vi "tdoa.vi"() -> ()   [LabVIEW 2015]
uses:
  <vilib>/rvi/Emulation/niFpgaGetClockAttributes.vi
  <vilib>/rvi/Emulation/niFpgaSctlEmulationGetInTimedLoop.vi
  <vilib>/rvi/Emulation/niFpgaEmulationReportErrorSimple.vi
  <vilib>/rvi/DataTransferAndStorage/Container/Common/niFpgaContainerGetUniqueNameForEmu.vi
  <vilib>/rvi/DataTransferAndStorage/Container/Common/niFpgaContainerSetEmuInfo.vi
  <vilib>/rvi/eio/common/nirviEmuReportErrorAndStop.vi
  <vilib>/rvi/eio/common/nirviEmuTemplateMethod_errors.vi
  <vilib>/rvi/interface/RandomDataEmulation/niFpgaRandomDataHandleErrors.vi
  <vilib>/rvi/DataTransferAndStorage/Container/Common/niFpgaContainerExecOnDevCompGetState.vi
  <vilib>/rvi/Emulation/niFpgaEmulationIsFPGAContextNoSignature.vi
  <vilib>/rvi/errors/niFpgaSetErrorForExecOnDevCompSimple.vi
  <vilib>/rvi/FIFO/Fifo_Resource/nirvififoEmulationSetSize.vi
  <vilib>/rvi/FIFO/Fifo_Resource/nirviFifoEmulationQueueMgr.vi
  <instcachedir>/0/nirviFifoEmulationQueueMgr_E5CAEC123FF24DC58D834DCA3CDAA9B5.lvgen/nirviFifoEmulationQueueMgr_E5CAEC123FF24DC58D834DCA3CDAA9B5_010.vi
  <vilib>/rvi/FIFO/Fifo_Resource/nirvififoEmulationDetermineInputValidOut.vi
  <vilib>/rvi/FIFO/Fifo_Resource/nirvififoEmulationCreateLock.vi
  <vilib>/rvi/Emulation/niFpgaProcessEmulError.vi
  <vilib>/rvi/FIFO/Fifo_Resource/nirvififoEmulationObtainLock.vi
  <vilib>/rvi/FIFO/Fifo_Resource/nirvififoEmulationReleaseLock.vi
  <vilib>/rvi/occurrence/nirviWaitOnOccurrenceBase.vi
  <vilib>/rvi/errors/nirviReportUnexpectedCaseInternalError.vi
  <vilib>/rvi/errors/nirviReportUnexpectedCaseInternalError (U32).vi
  <vilib>/Utility/error.llb/Clear Errors.vi
  <instcachedir>/0/nirviFifoEmulationQueueMgr_E5CAEC123FF24DC58D834DCA3CDAA9B5.lvgen/nirviFifoEmulationQueueMgr_E5CAEC123FF24DC58D834DCA3CDAA9B5_011.vi
  <vilib>/rvi/Emulation/niFpgaCriticalErrorInLSC.vi
  <vilib>/rvi/Memory/Memory_Emulation/niFpgaMemoryEmulationCacheClearOnFirstRun.vi
  <vilib>/rvi/Memory/Memory_Emulation/nirvimemoryEmulationManagerCache_MakeExclusive.vi
  <vilib>/rvi/Memory/Memory_Emulation/niFpgaMemoryEmulationValidateCache.vi
  <vilib>/rvi/Memory/Memory_Emulation/nirvimemoryEmulationManagerCache_InsertValue.vi
  <vilib>/rvi/Memory/Memory_Emulation/nirvimemoryEmulationManagerCache_ReleaseExclusive.vi
  <vilib>/rvi/Memory/Memory_Emulation/nirvimemoryEmulationManagerCache_GetValue.vi
  <vilib>/rvi/Memory/Memory_Emulation/nirvimemoryEmulationManagerCache_SetValue.vi
  <vilib>/rvi/Emulation/niFpgaSctlEmulationResourceMgr.vi
  <vilib>/rvi/LocalResourceManager/LocalResourceManager.xnode
  <vilib>/eio/EIONode/EIONode.xnode
  <vilib>/rvi/DataTransferAndStorage/Container/XNode/niFpgaContainer.xnode
  <vilib>/rvi/interface/RandomDataEmulation/nirviRandomDataFpgaReadWriteTemplate.vi
  <vilib>/rvi/FIFO/Fifo_Resource/niFpgaFifoEmulationRefIn.vi
  <vilib>/rvi/Memory/Memory_Emulation/niFpgaMemoryEmulationRefIn.vi
panel:
  out "xcorr1":fxp<+/-,32,30>
  out "xcorr1":fxp<+/-,32,30>
  out "Numeric 3":i32
  out "Numeric 2":i32
  out "Numeric":i32
  out "xcorr0":fxp<+/-,32,30>
  out "tdoa0":i32
  out "tdoa1":i32
  out "tdoa2":i32
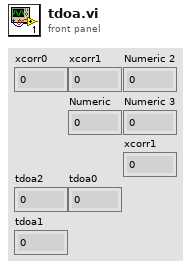
[diagram p1: front panel]
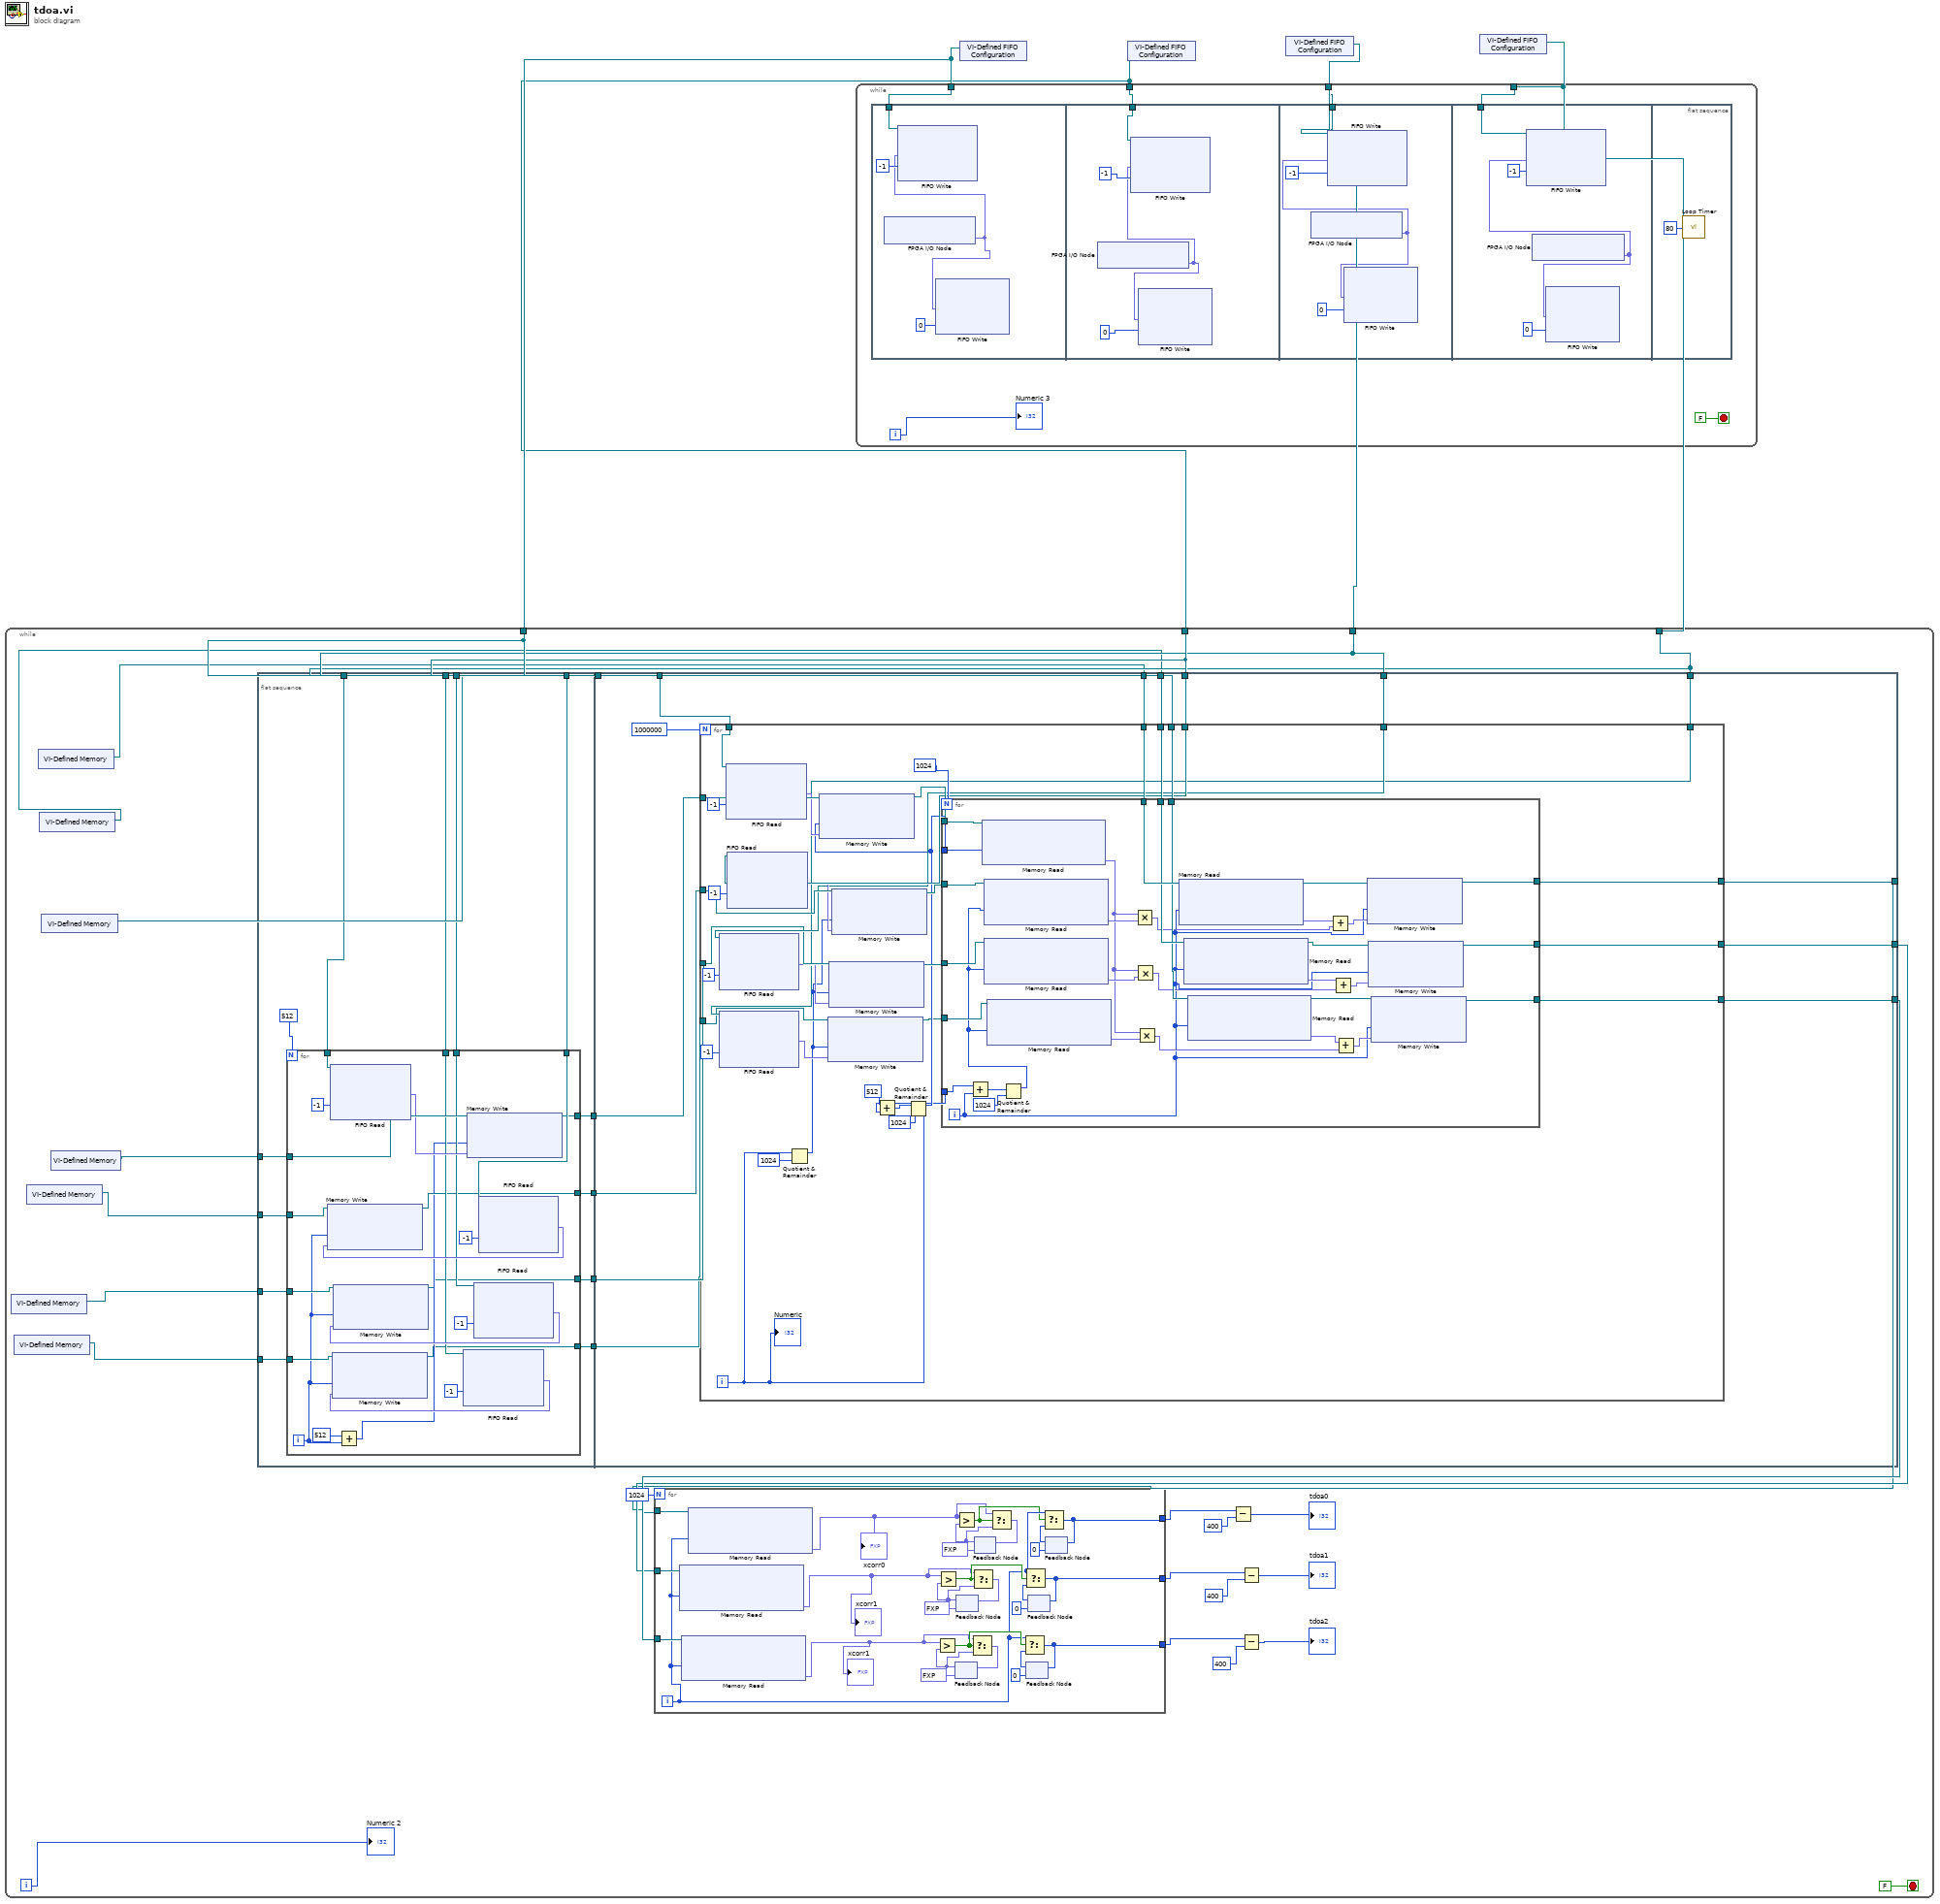
[diagram p0: block diagram]
diagram:
  n1 = xnode "VI-Defined FIFO Configuration"() -> ("FIFO Out"=w4:refnum<k21>)
  n2 = xnode "VI-Defined FIFO Configuration"() -> ("FIFO Out"=w3:refnum<k21>)
  n3 = xnode "VI-Defined FIFO Configuration"() -> ("FIFO Out"=w1:refnum<k21>)
  n4 = xnode "VI-Defined FIFO Configuration"() -> ("FIFO Out"=w2:refnum<k21>)
  n5 = while {
    tunnel: w1 -> [w30]
    tunnel: w2 -> [w29]
    tunnel: w4 -> [w33]
    tunnel: w3 -> [w31]
    i -> [w8]
    stop <- FALSE stop-if-true
    n6 = xnode "VI-Defined Memory"() -> ("Memory Out"=w6:refnum<k21>)
    n7 = xnode "VI-Defined Memory"() -> ("Memory Out"=w7:refnum<k21>)
    n8 = xnode "VI-Defined Memory"() -> ("Memory Out"=w5:refnum<k21>)
    n9 = xnode "VI-Defined Memory"() -> ("Memory Out"=w24:refnum<k21>)
    n10 = xnode "VI-Defined Memory"() -> ("Memory Out"=w23:refnum<k21>)
    n11 = xnode "VI-Defined Memory"() -> ("Memory Out"=w22:refnum<k21>)
    n12 = xnode "VI-Defined Memory"() -> ("Memory Out"=w32:refnum<k21>)
    n13 = flat-sequence {
      tunnel: w33 -> [w73]
      tunnel: w32 -> [w75]
      tunnel: w5 -> [w72]
      tunnel: w31 -> [w71]
      tunnel: w6 -> [w70]
      tunnel: w30 -> [w69]
      tunnel: w7 -> [w68]
      tunnel: w29 -> [w67]
      tunnel: [w66] -> w28
      tunnel: [w65] -> w27
      tunnel: [w64] -> w26
      tunnel: [w63] -> w25
      tunnel: w30 -> [w113]
      tunnel: w29 -> [w112]
      tunnel: w33 -> [w110]
      tunnel: w31 -> [w109]
      tunnel: w28 -> [w108]
      tunnel: w27 -> [w107]
      tunnel: w26 -> [w106]
      tunnel: w25 -> [w105]
      tunnel: w24 -> [w104]
      tunnel: w23 -> [w103]
      tunnel: w22 -> [w102]
      tunnel: [w101] -> w18
      tunnel: [w100] -> w17
      tunnel: [w99] -> w16
      frame #0 {
        n14 = for {
          N: 512 -> [_]
          tunnel: w75 -> [w98]
          tunnel: w73 -> [w97]
          tunnel: w72 -> [w94]
          tunnel: w71 -> [w92]
          tunnel: w70 -> [w89]
          tunnel: w69 -> [w88]
          tunnel: w68 -> [w85]
          tunnel: w67 -> [w84]
          tunnel: [w81] -> w66
          tunnel: [w80] -> w65
          tunnel: [w77] -> w64
          tunnel: [w76] -> w63
          i -> [w78]
          n15 = xnode ("FIFO Read")("Timeout"=-1, "FIFO In"=w97) -> ("Element"=w95:fxp<+/-,16,16>)  [unwired: 2 out]
          n16 = Add(x=512, y=w78) -> (x+y=w79:i32)
          n17 = xnode ("FIFO Read")("Timeout"=-1, "FIFO In"=w84) -> ("Element"=w83:fxp<+/-,32,16>)  [unwired: 2 out]
          n18 = xnode ("Memory Write")("Address"=w78, "Data"=w83, "Memory In"=w85) -> ("Memory Out"=w76:refnum<k21>)
          n19 = xnode ("Memory Write")("Address"=w79, "Data"=w95, "Memory In"=w98) -> ("Memory Out"=w81:refnum<k21>)
          n20 = xnode ("FIFO Read")("Timeout"=-1, "FIFO In"=w88) -> ("Element"=w87:fxp<+/-,32,16>)  [unwired: 2 out]
          n21 = xnode ("Memory Write")("Address"=w78, "Data"=w87, "Memory In"=w89) -> ("Memory Out"=w77:refnum<k21>)
          n22 = xnode ("FIFO Read")("Timeout"=-1, "FIFO In"=w92) -> ("Element"=w91:fxp<+/-,32,16>)  [unwired: 2 out]
          n23 = xnode ("Memory Write")("Address"=w78, "Data"=w91, "Memory In"=w94) -> ("Memory Out"=w80:refnum<k21>)
        }
      }
      frame #1 {
        n24 = for {
          N: 1000000 -> [_]
          tunnel: w113 -> [w131]
          tunnel: w112 -> [w124]
          tunnel: w110 -> [w138]
          tunnel: w109 -> [w135]
          tunnel: w108 -> [w140]
          tunnel: w107 -> [w134]
          tunnel: w106 -> [w128]
          tunnel: w105 -> [w123]
          tunnel: w104 -> [w143]
          tunnel: w103 -> [w142]
          tunnel: w102 -> [w141]
          tunnel: [w117] -> w101
          tunnel: [w116] -> w100
          tunnel: [w115] -> w99
          i -> [w114]
          n25 = xnode ("FIFO Read")("Timeout"=-1, "FIFO In"=w131) -> ("Element"=w125:fxp<+/-,32,16>)  [unwired: 2 out]
          n26 = xnode ("FIFO Read")("Timeout"=-1, "FIFO In"=w124) -> ("Element"=w121:fxp<+/-,32,16>)  [unwired: 2 out]
          n27 = xnode ("FIFO Read")("Timeout"=-1, "FIFO In"=w138) -> ("Element"=w136:fxp<+/-,16,16>)  [unwired: 2 out]
          n28 = xnode ("FIFO Read")("Timeout"=-1, "FIFO In"=w135) -> ("Element"=w132:fxp<+/-,32,16>)  [unwired: 2 out]
          n29 = Quotient & Remainder(x=w114, y=1024) -> (x-y*floor(x/y)=w118:i32)  [unwired: 1 out]
          n30 = xnode ("Memory Write")("Address"=w118, "Data"=w121, "Memory In"=w123) -> ("Memory Out"=w122:refnum<k21>)
          n31 = xnode ("Memory Write")("Address"=w118, "Data"=w125, "Memory In"=w128) -> ("Memory Out"=w127:refnum<k21>)
          n32 = xnode ("Memory Write")("Address"=w118, "Data"=w132, "Memory In"=w134) -> ("Memory Out"=w133:refnum<k21>)
          n33 = Add(x=512, y=w114) -> (x+y=w145:i32)
          n34 = Quotient & Remainder(x=w145, y=1024) -> (x-y*floor(x/y)=w126:i32)  [unwired: 1 out]
          n35 = xnode ("Memory Write")("Address"=w126, "Data"=w136, "Memory In"=w140) -> ("Memory Out"=w139:refnum<k21>)
          n36 = for {
            N: 1024 -> [_]
            tunnel: w139 -> [w179]
            tunnel: w133 -> [w178]
            tunnel: w114 -> [w176]
            tunnel: w126 -> [w177]
            tunnel: w127 -> [w173]
            tunnel: w122 -> [w172]
            tunnel: w143 -> [w166]
            tunnel: w142 -> [w165]
            tunnel: w141 -> [w164]
            tunnel: [w150] -> w115
            tunnel: [w149] -> w116
            tunnel: [w148] -> w117
            i -> [w151]
            n37 = Add(x=w176, y=w151) -> (x+y=w175:i32)
            n38 = xnode ("Memory Read")("Address"=w177, "Memory In"=w179) -> ("Data"=w167:fxp<+/-,32,16>)  [unwired: 1 out]
            n39 = Quotient & Remainder(x=w175, y=1024) -> (x-y*floor(x/y)=w171:i32)  [unwired: 1 out]
            n40 = xnode ("Memory Read")("Address"=w171, "Memory In"=w178) -> ("Data"=w168:fxp<+/-,32,16>)  [unwired: 1 out]
            n41 = xnode ("Memory Read")("Address"=w171, "Memory In"=w173) -> ("Data"=w169:fxp<+/-,32,16>)  [unwired: 1 out]
            n42 = xnode ("Memory Read")("Address"=w171, "Memory In"=w172) -> ("Data"=w170:fxp<+/-,32,16>)  [unwired: 1 out]
            n43 = Multiply(x=w167, y=w168) -> (x*y=w162:fxp<+/-,64,32>)
            n44 = Multiply(x=w167, y=w169) -> (x*y=w160:fxp<+/-,64,32>)
            n45 = Multiply(x=w167, y=w170) -> (x*y=w158:fxp<+/-,64,32>)
            n46 = xnode ("Memory Read")("Address"=w151, "Memory In"=w166) -> ("Data"=w163:fxp<+/-,64,32>, "Memory Out"=w157:refnum<k21>)
            n47 = xnode ("Memory Read")("Address"=w151, "Memory In"=w165) -> ("Data"=w161:fxp<+/-,64,32>, "Memory Out"=w156:refnum<k21>)
            n48 = xnode ("Memory Read")("Address"=w151, "Memory In"=w164) -> ("Data"=w159:fxp<+/-,64,32>, "Memory Out"=w155:refnum<k21>)
            n49 = Add(x=w163, y=w162) -> (x+y=w152:fxp<+/-,64,33>)
            n50 = Add(x=w161, y=w160) -> (x+y=w153:fxp<+/-,64,33>)
            n51 = Add(x=w159, y=w158) -> (x+y=w154:fxp<+/-,64,33>)
            n52 = xnode ("Memory Write")("Address"=w151, "Data"=w152, "Memory In"=w157) -> ("Memory Out"=w150:refnum<k21>)
            n53 = xnode ("Memory Write")("Address"=w151, "Data"=w153, "Memory In"=w156) -> ("Memory Out"=w149:refnum<k21>)
            n54 = xnode ("Memory Write")("Address"=w151, "Data"=w154, "Memory In"=w155) -> ("Memory Out"=w148:refnum<k21>)
          }
          "Numeric" <- w114
        }
      }
    }
    n55 = for {
      N: 1024 -> [_]
      tunnel: [w51] -> w10
      tunnel: [w50] -> w11
      tunnel: [w43] -> w12
      tunnel: w18 -> [w40]
      tunnel: w17 -> [w41]
      tunnel: w16 -> [w42]
      i -> [w39]
      n56 = xnode ("Memory Read")("Address"=w39, "Memory In"=w41) -> ("Data"=w35:fxp<+/-,64,32>)  [unwired: 1 out]
      "xcorr1" <- w35
      n57 = xnode ("Memory Read")("Address"=w39, "Memory In"=w40) -> ("Data"=w36:fxp<+/-,64,32>)  [unwired: 1 out]
      "xcorr1" <- w36
      n58 = xnode ("Memory Read")("Address"=w39, "Memory In"=w42) -> ("Data"=w37:fxp<+/-,64,32>)  [unwired: 1 out]
      "xcorr0" <- w37
      n59 = feedback #1(fxp<+/-,64,60> -1000.0 ("element")) -> (w45:fxp<+/-,64,60>)
      n60 = Greater?(x=w36, y=w45) -> (0:w47:bool)
      n61 = feedback #2(fxp<+/-,64,60> -1000.0 ("element")) -> (w56:fxp<+/-,64,60>)
      n62 = Greater?(x=w35, y=w56) -> (0:w54:bool)
      n63 = Select(t=w36, s=w47, f=w45) -> (s? t:f=w44:fxp<+/-,64,60>)
      n64 = feedback-in #1(w44) -> ()
      n65 = Select(t=w35, s=w54, f=w56) -> (s? t:f=w57:fxp<+/-,64,60>)
      n66 = feedback-in #2(w57) -> ()
      n67 = feedback #3(fxp<+/-,64,60> -1000.0 ("element")) -> (w61:fxp<+/-,64,60>)
      n68 = Greater?(x=w37, y=w61) -> (0:w38:bool)
      n69 = Select(t=w37, s=w38, f=w61) -> (s? t:f=w62:fxp<+/-,64,60>)
      n70 = feedback-in #3(w62) -> ()
      n71 = feedback #4(0) -> (w48:i32)
      n72 = Select(t=w39, s=w47, f=w48) -> (s? t:f=w43:i32)
      n73 = feedback-in #4(w43) -> ()
      n74 = feedback #5(0) -> (w53:i32)
      n75 = Select(t=w39, s=w54, f=w53) -> (s? t:f=w50:i32)
      n76 = feedback-in #5(w50) -> ()
      n77 = feedback #6(0) -> (w59:i32)
      n78 = Select(t=w39, s=w38, f=w59) -> (s? t:f=w51:i32)
      n79 = feedback-in #6(w51) -> ()
    }
    n80 = Subtract(x=w10, y=i16 400 ("x")) -> (x-y=→"tdoa0":i32)
    n81 = Subtract(x=w11, y=i16 400 ("x")) -> (x-y=→"tdoa1":i32)
    n82 = Subtract(x=w12, y=i16 400 ("x")) -> (x-y=→"tdoa2":i32)
    "Numeric 2" <- w8
  }
  n83 = while {
    tunnel: w4 -> [w184]
    tunnel: w3 -> [w181]
    tunnel: w1 -> [w182]
    tunnel: w2 -> [w183]
    i -> [w180]
    stop <- FALSE stop-if-true
    n84 = flat-sequence {
      tunnel: w184 -> [w189]
      tunnel: w181 -> [w192]
      tunnel: w182 -> [w197]
      tunnel: w183 -> [w200]
      frame #0 {
        n85 = xnode "FPGA I/O Node"() -> ("Connector0/AI0"=w186:fxp<+/-,27,5>)  [unwired: 1 in, 1 out]
        n86 = xnode ("FIFO Write")("Element"=w186, "Timeout"=-1, "FIFO In"=w189) -> ()  [unwired: 2 out]
        n87 = xnode ("FIFO Write")("Element"=w186, "Timeout"=0) -> ()  [unwired: 1 in, 2 out]
      }
      frame #1 {
        n88 = xnode "FPGA I/O Node"() -> ("Connector0/AI1"=w190:fxp<+/-,27,5>)  [unwired: 1 in, 1 out]
        n89 = xnode ("FIFO Write")("Element"=w190, "Timeout"=-1, "FIFO In"=w192) -> ()  [unwired: 2 out]
        n90 = xnode ("FIFO Write")("Element"=w190, "Timeout"=0) -> ()  [unwired: 1 in, 2 out]
      }
      frame #2 {
        n91 = xnode "FPGA I/O Node"() -> ("Connector0/AI2"=w195:fxp<+/-,27,5>)  [unwired: 1 in, 1 out]
        n92 = xnode ("FIFO Write")("Element"=w195, "Timeout"=-1, "FIFO In"=w197) -> ()  [unwired: 2 out]
        n93 = xnode ("FIFO Write")("Element"=w195, "Timeout"=0) -> ()  [unwired: 1 in, 2 out]
      }
      frame #3 {
        n94 = xnode "FPGA I/O Node"() -> ("Connector0/AI3"=w198:fxp<+/-,27,5>)  [unwired: 1 in, 1 out]
        n95 = xnode ("FIFO Write")("Element"=w198, "Timeout"=-1, "FIFO In"=w200) -> ()  [unwired: 2 out]
        n96 = xnode ("FIFO Write")("Element"=w198, "Timeout"=0) -> ()  [unwired: 1 in, 2 out]
      }
      frame #4 {
        n97 = call "Loop Timer"("Count(Ticks)"=u32 80) -> ()  [unwired: 1 out]
      }
    }
    "Numeric 3" <- w180
  }
